vi "Alp Proj Inquire.vi"(8 "error in (no error)":errorcluster, 9 "UserVarPtr":i32, 10 "InquireType":i32, 11 "DeviceId":u32) -> (0 "error out":errorcluster, 1 "UserVarPtr out":i32, 3 "function return":i32)   [LabVIEW 2013, in "alpD41.lvlib"]
uses:
  <userlib>/alpD41/alpD41.lvlib
  <userlib>/alpD41/alpD41.dll
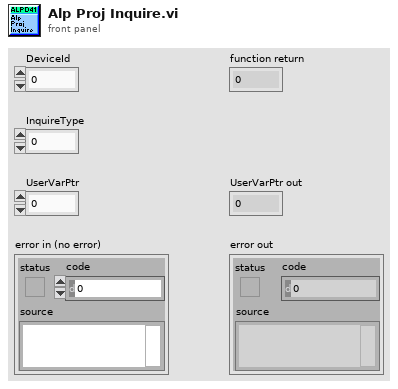
[diagram p1: front panel]
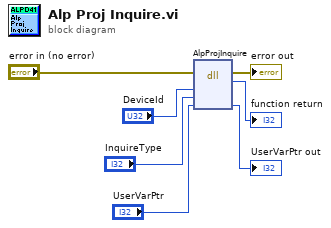
[diagram p0: block diagram]
diagram:
  n1 = dll-call lib="C:/Program Files (x86)/National Instruments/LabVIEW 2013/user.lib/alpD41/alpD41.*" fn="AlpProjInquire"(error in="error in (no error)", "DeviceId"="DeviceId", "InquireType"="InquireType", "UserVarPtr"="UserVarPtr") -> (error out=→"error out":errorcluster, →"function return":i32, "UserVarPtr"=→"UserVarPtr out":i32)  [unwired: 4 in, 1 out]
